vi "batch_processor_query.vi"(8 "error in (no error)":errorcluster, 9 "Live Run?":bool, 10 "Small?":bool, 11 "Update Error files?":bool) -> (0 "error out":errorcluster, 1 "Old Processing":bool, 2 "Total Events":i32, 3 "BP Array":T1[](array[typedef]) {"File Location" items=["Unknown"=-1, "Storage"=0, "Processing"=1, "Unmerged"=2]})   [LabVIEW 2013]
doc: "Specifically for batch processing purposes. Searches the database for particles with file_location = \"0\", or Processing. \"Live Run\" makes this program only return events from the most recent experiment. Update Error files returns all dust events for which file_location is less than 0. Each particle found is returned as a cluster of id_dust_event, pelletron_high_voltage (simple voltage on the small acc), id_experiment_settings, file_location, and dust_density."
uses:
  <userlib>/Accelerator/User Interface/Controls/bp_cluster.ctl
  <userlib>/Accelerator/User Interface/Controls/File_location.ctl
  <userlib>/_OpenG.lib/array/array.llb/Empty 2D Array (Variant)__ogtk.vi
  <vilib>/addons/database/_DB Variant To Data/Database Variant To Data.xnode
panel:
  out "Count Events Syntax":string
  out "SQL Query Syntax":string
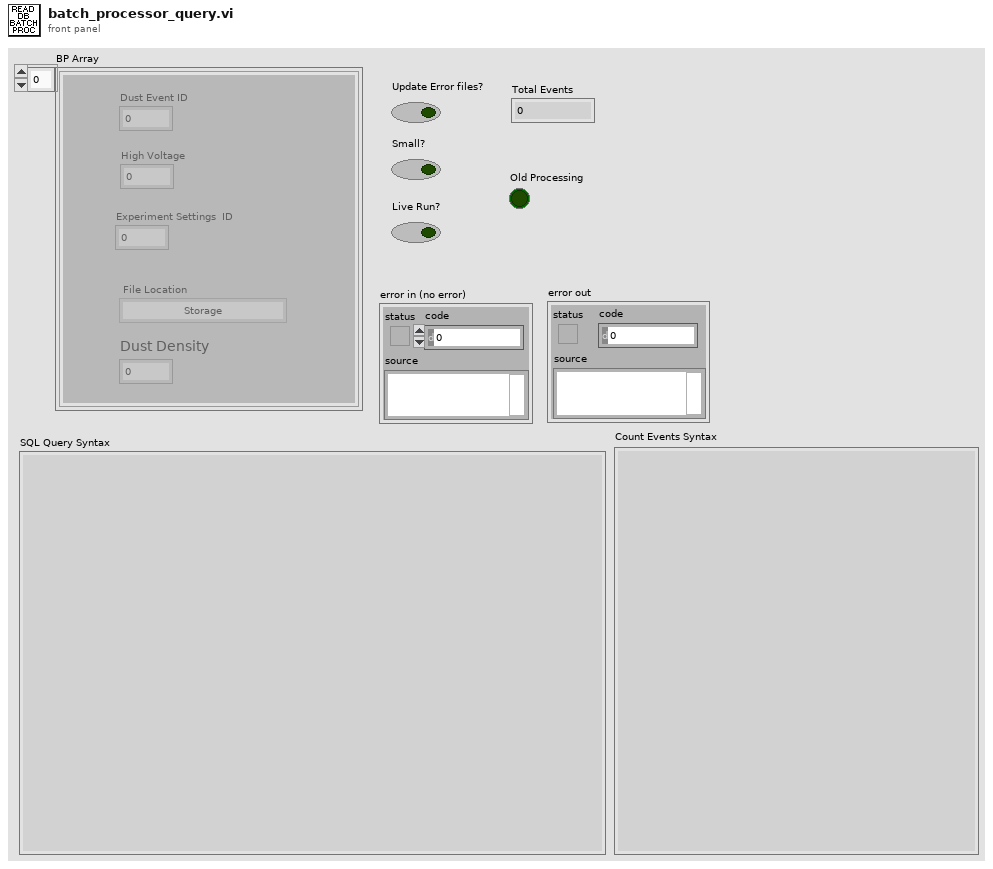
[diagram p1: front panel]
types:
  T1 = typedef "bp_cluster.ctl" = cluster{"Dust Event ID":i64, "High Voltage":sgl, "Experiment Settings  ID":i64, "File Location":T2, "Dust Density":dbl}
  T2 = typedef "File_location.ctl" = i8
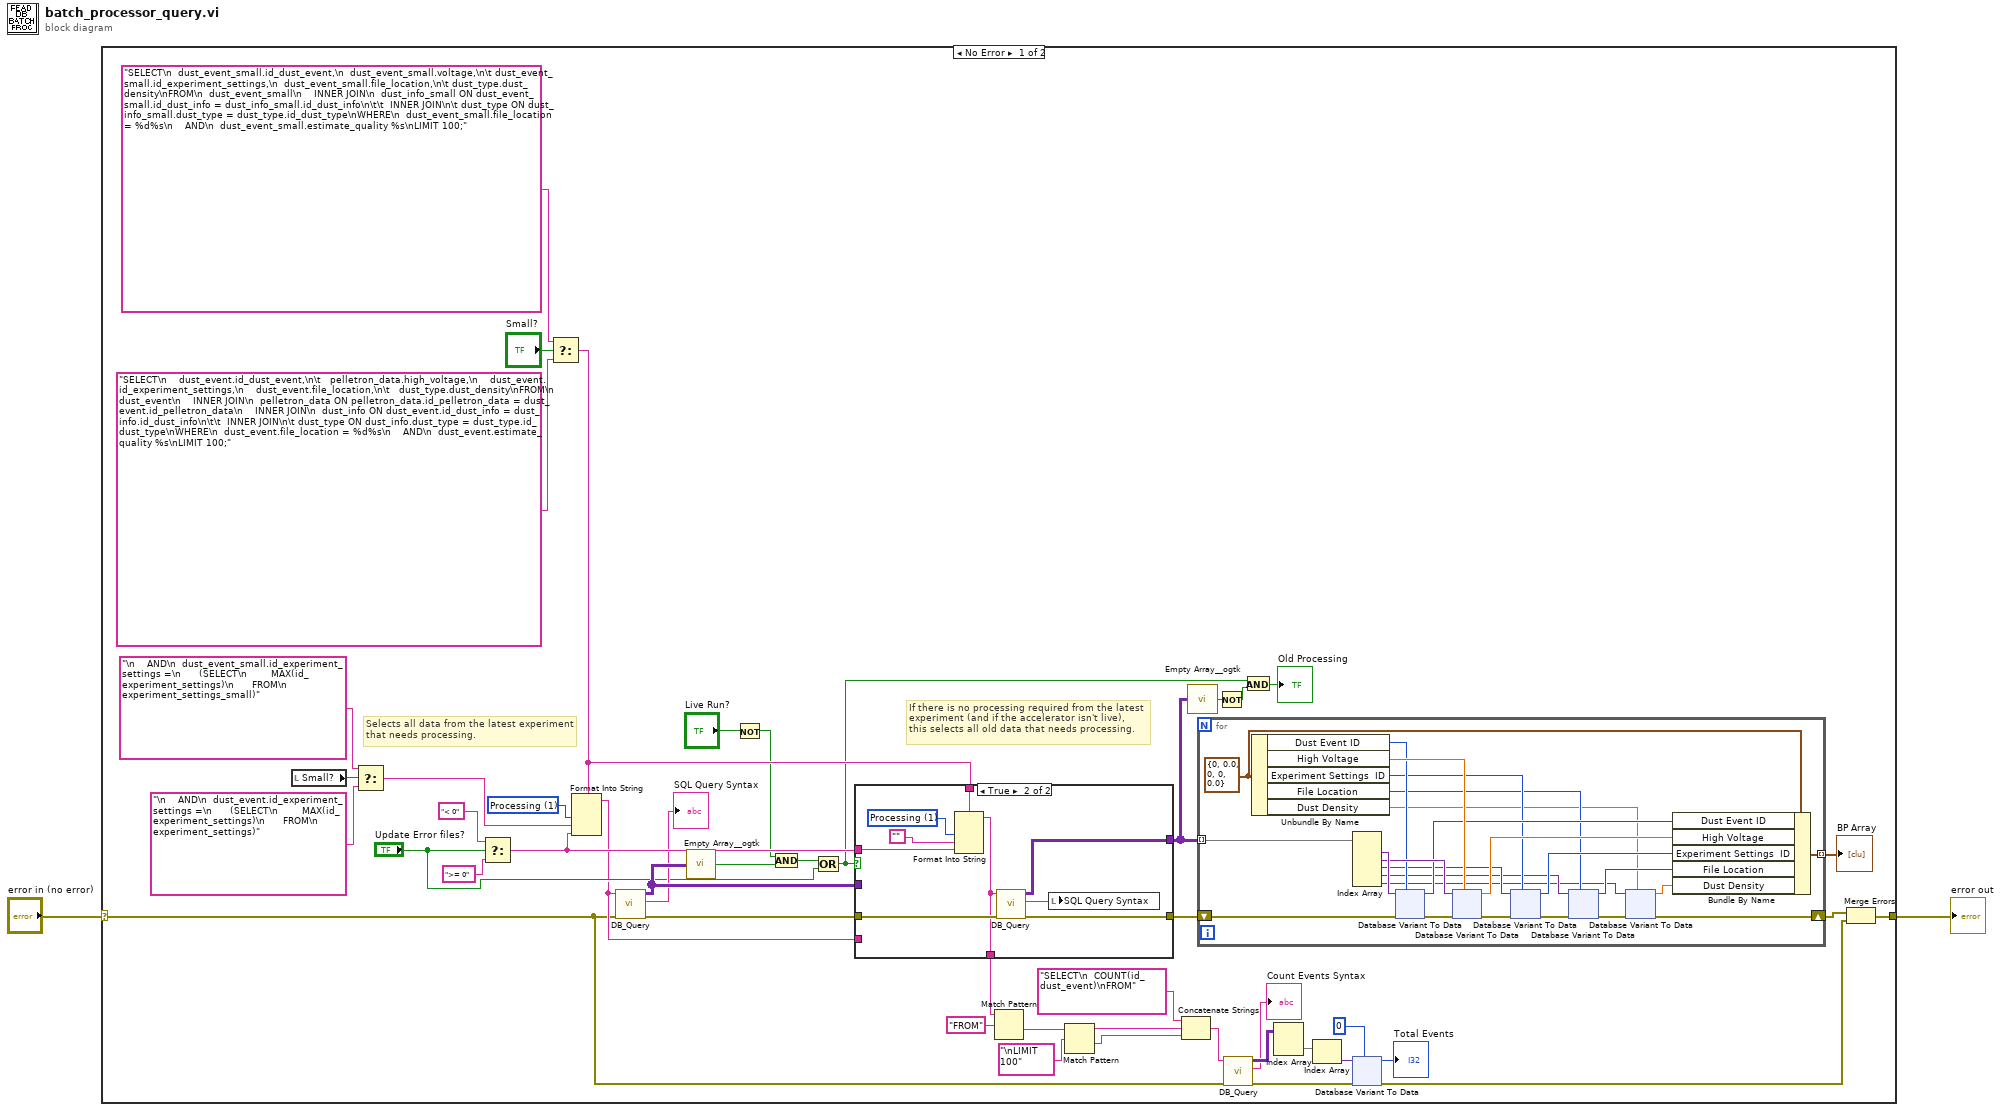
[diagram p0: block diagram]
diagram:
  n1 = case shown="No Error" "error in (no error)" {
    selector: "error in (no error)" -> [w21 w278]
    tunnel: [w13 w278] -> w1
    frame No Error {
      w43 = T2 1 items=["Unknown"=-1, "Storage"=0, "Processing"=1, "Unmerged"=2] ("File Location")
      # "If there is no processing required from the latest\nexperiment (and if the accelerator isn't live),\nthis selects all old data that needs processing."
      # "Selects all data from the latest experiment\nthat needs processing."
      n2 = local read "Small?"() -> (w37:bool)
      n3 = Select(t="\n    AND\n  dust_event_small.id_experiment_settings =\n      (SELECT\n        MAX(id_experiment_settings)\n      FROM\n        experiment_settings_small)" ("input 2"), s=w37, f="\n    AND\n  dust_event.id_experiment_settings =\n      (SELECT\n        MAX(id_experiment_settings)\n      FROM\n        experiment_settings)" ("input 2")) -> (s? t:f=w36:string)
      n4 = Select(t="< 0", s="Update Error files?", f=">= 0") -> (s? t:f=w42:string)
      n5 = Select(t="SELECT\n  dust_event_small.id_dust_event,\n  dust_event_small.voltage,\n\t dust_event_small.id_experiment_settings,\n  dust_event_small.file_location,\n\t dust_type.dust_density\nFROM\n  dust_event_small\n    INNER JOIN\n  dust_info_small ON dust_event_small.id_dust_info = dust_info_small.id_dust_info\n\t\t  INNER JOIN\n\t dust_type ON dust_info_small.dust_type = dust_type.id_dust_type\nWHERE\n  dust_event_small.file_location = %d%s\n    AND\n  dust_event_small.estimate_quality %s\nLIMIT 100;" ("string"), s="Small?", f="SELECT\n    dust_event.id_dust_event,\n\t   pelletron_data.high_voltage,\n    dust_event.id_experiment_settings,\n    dust_event.file_location,\n\t   dust_type.dust_density\nFROM\n  dust_event\n    INNER JOIN\n  pelletron_data ON pelletron_data.id_pelletron_data = dust_event.id_pelletron_data\n    INNER JOIN\n  dust_info ON dust_event.id_dust_info = dust_info.id_dust_info\n\t\t  INNER JOIN\n\t dust_type ON dust_info.dust_type = dust_type.id_dust_type\nWHERE\n  dust_event.file_location = %d%s\n    AND\n  dust_event.estimate_quality %s\nLIMIT 100;" ("string")) -> (s? t:f=w41:string)
      n6 = Format Into String(format string=w41, w43, w36, w42) -> (resulting string=w22:string)  [unwired: 2 in, 1 out]
      n7 = call <userlib>:"DB_Query.vi"("error in (no error)"=w21, "Parameterized Query"=w22) -> ("error out"=w28:errorcluster, "Query in Standard Format"=→"SQL Query Syntax":string, "Results"=w27:variant[][])  [unwired: 7 in]
      n8 = call-poly <userlib>:"Empty Array__ogtk.vi"("Array"=w27) -> ("Empty Array?"=w33:bool)  [unwired: 8 in]
      n9 = Not(x="Live Run?") -> (.not. x?=w34:bool)
      n10 = And(x=w34, y=w33) -> (x .and. y?=w24:bool)
      n11 = Or(x=w24, y="Update Error files?") -> (x .or. y?=w25:bool)
      n12 = case shown="True" w25 {
        tunnel: [w84 w87] -> w29
        tunnel: w27 -> [w84 _]
        tunnel: w42 -> [_ w93]
        tunnel: w41 -> [_ w90]
        tunnel: [w83 w86] -> w40
        tunnel: w28 -> [w83 w89]
        tunnel: [w82 w85] -> w10
        tunnel: w22 -> [w82 _]
        frame False {
        }
        frame True {
          w91 = T2 1 items=["Unknown"=-1, "Storage"=0, "Processing"=1, "Unmerged"=2] ("input 1")
          n13 = Format Into String(format string=w90, w91, "", w93) -> (resulting string=w85:string)  [unwired: 2 in, 1 out]
          n14 = call <userlib>:"DB_Query.vi"("error in (no error)"=w89, "Parameterized Query"=w85) -> ("error out"=w86:errorcluster, "Query in Standard Format"=w88:string, "Results"=w87:variant[][])  [unwired: 7 in]
          n15 = local write "SQL Query Syntax"(w88) -> ()
        }
      }
      n16 = Match Pattern(string=w10, regular expression="FROM") -> (after substring=w8:string)  [unwired: 1 in, 3 out]
      n17 = Match Pattern(string=w8, regular expression="\nLIMIT 100") -> (before substring=w5:string, after substring=w4:string)  [unwired: 1 in, 2 out]
      n18 = Concatenate Strings("SELECT\n  COUNT(id_dust_event)\nFROM" ("input 1"), w5, w4) -> (w3:string)
      n19 = call-poly <userlib>:"Empty Array__ogtk.vi"("Array"=w29) -> ("Empty Array?"=w30:bool)  [unwired: 8 in]
      n20 = for {
        tunnel: w29 -> [w117] mode=indexing
        shift-right: [w114] -> w12
        shift-left: w40 -> [w116]
        tunnel: [w115] -> w49 mode=indexing
        w106 = T1 {"Dust Event ID"=0, "High Voltage"=0.0, "Experiment Settings  ID"=0, "File Location"=0, "Dust Density"=0.0} ("Batch Processing Cluster")
        n21 = Unbundle By Name(w106) -> ("Dust Event ID"=w108:i64, "High Voltage"=w109:sgl, "Experiment Settings  ID"=w104:i64, "File Location"=w99:T2, "Dust Density"=w96:dbl)
        n22 = Index Array(array=w117) -> (element #1=w113:variant, element #2=w112:variant, element #3=w105:variant, element #4=w101:variant, element #5=w95:variant)  [unwired: 5 in]
        n23 = xnode "Database Variant To Data"("database variant"=w113, "error in"=w116, "type"=w108) -> ("data"=w107:i64, "error out"=w111:errorcluster)
        n24 = xnode "Database Variant To Data"("database variant"=w112, "error in"=w111, "type"=w109) -> ("data"=w110:sgl, "error out"=w102:errorcluster)
        n25 = xnode "Database Variant To Data"("database variant"=w105, "error in"=w102, "type"=w104) -> ("data"=w103:i64, "error out"=w100:errorcluster)
        n26 = xnode "Database Variant To Data"("database variant"=w101, "error in (no error)"=w100, "type"=w99) -> ("data"=w98:T2, "error out"=w97:errorcluster)
        n27 = xnode "Database Variant To Data"("database variant"=w95, "error in"=w97, "type"=w96) -> ("data"=w94:dbl, "error out"=w114:errorcluster)
        n28 = Bundle By Name(cluster=w106, "Dust Event ID"=w107, "High Voltage"=w110, "Experiment Settings  ID"=w103, "File Location"=w98, "Dust Density"=w94) -> (w115:T1)
      }
      "BP Array" <- w49
      n29 = Not(x=w30) -> (.not. x?=w31:bool)
      n30 = call <userlib>:"DB_Query.vi"("error in (no error)"=w21, "Parameterized Query"=w3) -> ("error out"=w17:errorcluster, "Query in Standard Format"=→"Count Events Syntax":string, "Results"=w20:variant[][])  [unwired: 7 in]
      n31 = And(x=w25, y=w31) -> (x .and. y?=→"Old Processing":bool)
      n32 = Index Array(array=w20) -> (element=w19:variant[])  [unwired: 2 in]
      n33 = Index Array(array=w19) -> (element=w18:variant)  [unwired: 1 in]
      n34 = xnode "Database Variant To Data"("database variant"=w18, "error in (no error)"=w17, "type"=0 ("Total Events")) -> ("data"=→"Total Events":i32, "error out"=w11:errorcluster)
      n35 = Merge Errors(w12, w11) -> (w13:errorcluster)
    }
    frame Error {
    }
  }
  "error out" <- w1
